vi "Create Same Type Image.vi"(8 "error in (no error)":errorcluster, 9 "Name in":string, 10 "Image Dst":T1, 11 "Image Src":T1) -> (0 "error out":errorcluster, 1 "Name out":string, 3 "Image Dst":T1)   [LabVIEW 2021, in "Image.lvlib"]
uses:
  <vilib>/vision/Image Controls.llb/IMAQ Image.ctl
  Image.lvlib
panel:
  out "Message":string
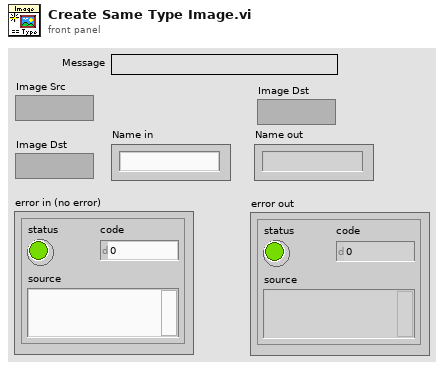
[diagram p1: front panel]
types:
  T1 = typedef "IMAQ Image.ctl" = refnum<image>
  T2 = typedef "Image Type" = u32
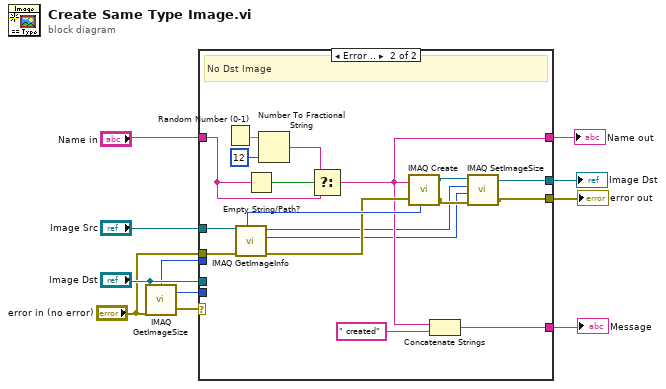
[diagram p0: block diagram]
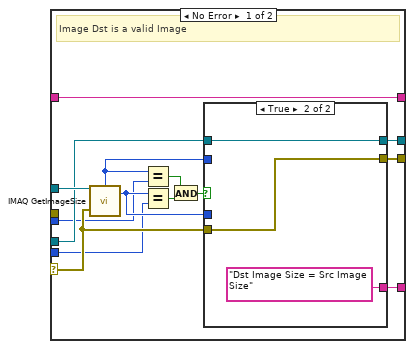
[diagram p2: hidden frame]
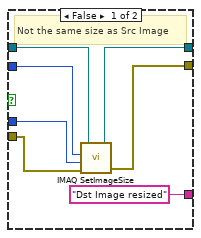
[diagram p3: hidden frame]
diagram:
  n1 = call "IMAQ GetImageSize"("Image"="Image Dst", "error in (no error)"="error in (no error)") -> ("Y Resolution"=w3:i32, "X Resolution"=w2:i32, "error out"=w4:errorcluster)  [unwired: 2 in]
  n2 = case shown="Error .." w4 {
    selector: w4 -> [w14 _]
    tunnel: "Image Src" -> [w25 w53]
    tunnel: "Name in" -> [w18 w46]
    tunnel: [w19 w39] -> w9
    tunnel: [w18 w45] -> w8
    tunnel: [w20 w38] -> w7
    tunnel: "Image Dst" -> [w21 _]
    tunnel: [w15 w43] -> w6
    tunnel: w3 -> [w13 _]
    tunnel: w2 -> [w12 _]
    tunnel: "error in (no error)" -> [_ w42]
    frame No Error {
      # "Image Dst is a valid Image"
      n3 = call "IMAQ GetImageSize"("Image"=w25, "error in (no error)"=w14) -> ("Y Resolution"=w16:i32, "X Resolution"=w17:i32)  [unwired: 2 in, 1 out]
      n4 = Equal?(x=w17, y=w12) -> (x = y?=w24:bool)
      n5 = Equal?(x=w16, y=w13) -> (x = y?=w23:bool)
      n6 = And(x=w24, y=w23) -> (x .and. y?=w22:bool)
      n7 = case shown="True" w22 {
        tunnel: w21 -> [w32 w35]
        tunnel: [w31 w35] -> w20
        tunnel: [w30 w33] -> w19
        tunnel: w17 -> [w29 _]
        tunnel: w16 -> [w28 _]
        tunnel: w14 -> [w27 w33]
        tunnel: ["Dst Image resized" "Dst Image Size = Src Image Size"] -> w15
        frame False {
          # "Not the same size as Src Image"
          n8 = call "IMAQ SetImageSize"("error in (no error)"=w27, "Y Resolution"=w28, "X Resolution"=w29, "Image"=w32) -> ("error out"=w30:errorcluster, "Image Out"=w31:T1)  [unwired: 1 in]
        }
        frame True {
        }
      }
    }
    frame Error {
      # "No Dst Image"
      n9 = Random Number (0-1)() -> (number: 0 to 1=w49:dbl)
      n10 = call "IMAQ GetImageInfo"("error in (no error)"=w42, "Image"=w53) -> ("error out"=w51:errorcluster, "Y Resolution"=w36:i32, "X Resolution"=w37:i32, "Image Type"=w52:T2)  [unwired: 2 in, 4 out]
      n11 = Empty String/Path?(string/path=w46) -> (empty?=w50:bool)
      n12 = Number To Fractional String(number=w49, precision (6)=i16 12) -> (F-format string=w47:string)  [unwired: 2 in]
      n13 = Select(t=w47, s=w50, f=w46) -> (s? t:f=w45:string)
      n14 = call "IMAQ Create"("Image Name"=w45, "Image Type"=w52, "error in (no error)"=w51) -> ("New Image"=w41:T1, "error out"=w40:errorcluster)  [unwired: 2 in]
      n15 = Concatenate Strings(w45, " created" ("string")) -> (w43:string)
      n16 = call "IMAQ SetImageSize"("error in (no error)"=w40, "Y Resolution"=w36, "X Resolution"=w37, "Image"=w41) -> ("error out"=w39:errorcluster, "Image Out"=w38:T1)  [unwired: 1 in]
    }
  }
  "error out" <- w9
  "Image Dst" <- w7
  "Name out" <- w8
  "Message" <- w6
